vi "Parsing Error.vi"(7 "JSON":string, 8 "error in (no error)":errorcluster, 9 "Offset past match":i32=-1, 10 "Value start":i32=-1, 11 "State":T1) -> (0 "error out":errorcluster)   [LabVIEW 2015, in "JSONtext.lvlib"]
uses:
  JSONtext.lvlib
  Parsing State.ctl
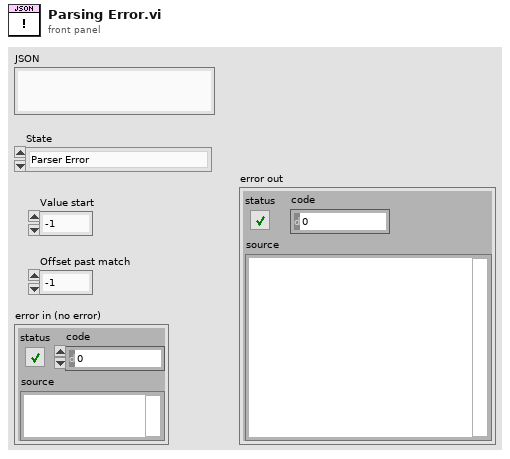
[diagram p1: front panel]
types:
  T1 = typedef "JSONtext.lvlib/Parsing State.ctl" = enum16{"Parser Error", "Object", "Array", "String", "Number/Other", "Leading Whitespace", "Object end", "Array end", "Value end"}
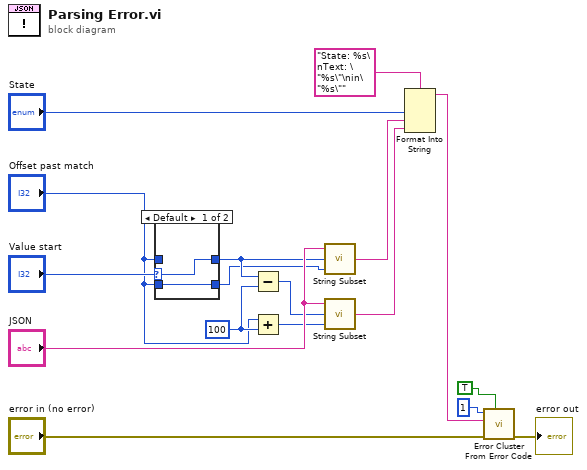
[diagram p0: block diagram]
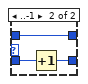
[diagram p2: hidden frame]
diagram:
  w8 = 100 ("y")
  n1 = case shown="Default" "Value start" {
    selector: "Value start" -> [w19 _]
    tunnel: [w19 w22] -> w4
    tunnel: "Offset past match" -> [_ w22]
    tunnel: "Offset past match" -> [w18 w20]
    tunnel: [w18 w21] -> w2
    frame Default {
    }
    frame ..-1 {
      n2 = Increment(x=w20) -> (x+1=w21:i32)
    }
  }
  n3 = Subtract(x=w4, y=w8) -> (x-y=w10:i32)
  n4 = Add(x="Offset past match", y=w8) -> (x+y=w7:i32)
  n5 = call "String Subset.vi"("Offset past End"=w2, "Start offset"=w4, "JSON"="JSON") -> ("substring"=w13:string)  [unwired: 2 in]
  n6 = call "String Subset.vi"("Offset past End"=w7, "Start offset"=w10, "JSON"="JSON") -> ("substring"=w9:string)  [unwired: 2 in]
  n7 = Format Into String(format string="State: %s\nText: \"%s\"\nin\"%s\"", "State", w13, w9) -> (resulting string=w16:string)  [unwired: 2 in, 1 out]
  n8 = call <vilib>:"Error Cluster From Error Code.vi"("show call chain? (False)"=TRUE, "error in (no error)"="error in (no error)", "error message (\"\")"=w16, "error code (0)"=1) -> ("error out"=→"error out":errorcluster)  [unwired: 5 in]
